vi "Save Report As PDF 2012 NIVerified.vi"(8 "error in (no error)":errorcluster, 10 "Data Set Name":string, 11 "Report file path":path=path "D:/Customer stuff/1944517 Tom Frei/test.xlsx") -> (0 "error out":errorcluster, 3 "Report Saved Path":path)   [LabVIEW 2020]
doc: "This VI demonstrates how to use ActiveX methods to save a Word or Excel report as a PDF."
uses:
  <vilib>/Utility/sysdir.llb/System Directory Type.ctl
  <vilib>/Utility/NIReport.llb/NI_report.lvclass
  <vilib>/Utility/NIReport.llb/Word/NI_Word.lvclass
  <vilib>/Utility/NIReport.llb/Excel/NI_Excel.lvclass
panel:
  # "Overview: Demonstrates how to use ActiveX methods to save a Word or Excel report as a PDF.  \nRequirements: LabVIEW 2012 (or compatible), Report Generation Toolkit\nInstructions: \n1. Browse for an existing Word or Excel document.\n2. Select the appropriate Report Type.\n3. Run the VI and it will save the document as a PDF as \"LabVIEW Save.pdf\" in the same folder as the original report."
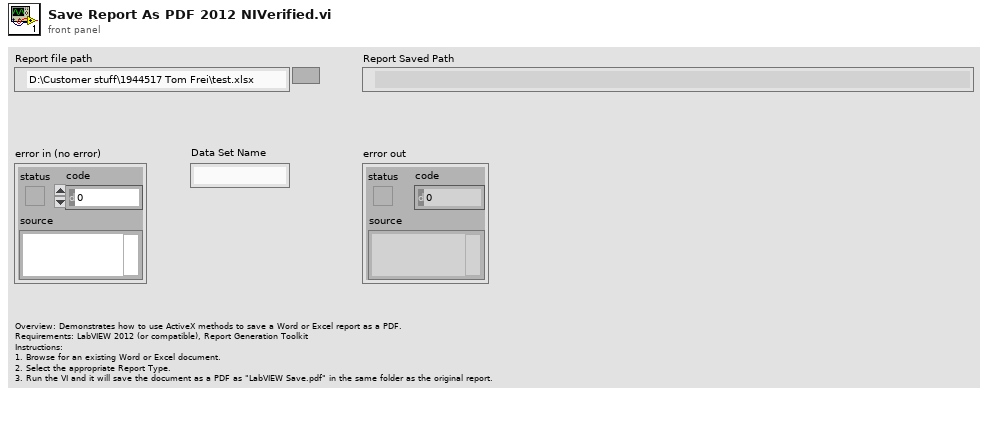
[diagram p1: front panel]
types:
  T1 = typedef "System Directory Type.ctl" = i32
  T2 = enum16{"Standard Report", "HTML", "Word", "Excel"}
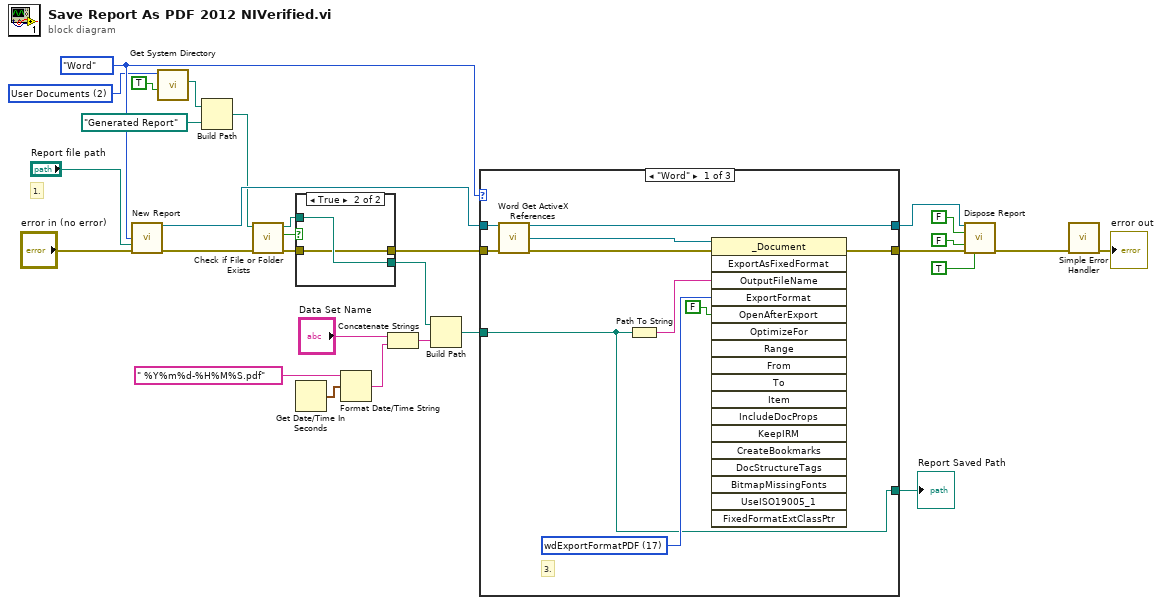
[diagram p0: block diagram]
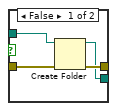
[diagram p2: hidden frame]
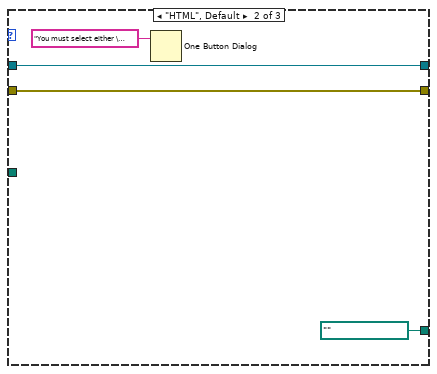
[diagram p3: hidden frame]
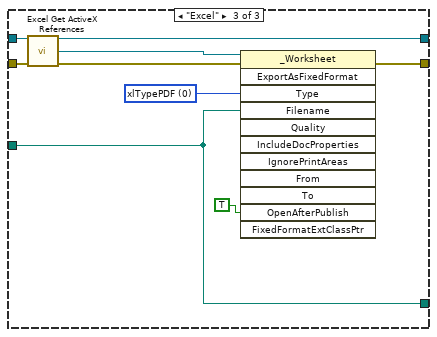
[diagram p4: hidden frame]
diagram:
  w21 = T1 2 items=["User Home"=0, "User Desktop"=1, "User Documents"=2, "User Application Data"=3, "User Preferences"=4, "User Temporary"=5, "Public Documents"=6, "Public Application Data"=7, "Public Preferences"=8, "Public Cache"=13, "System Core Libraries"=9, "System Installed Libraries"=10, "Application Files"=11, "Boot Volume Root"=12] ("system directory type")
  w27 = T2."Word" ("Report Type")
  # "1."
  n1 = call <vilib>:"New Report.vi"("report type"=w27, "template (empty)"="Report file path", "error in (no error)"="error in (no error)") -> ("report out"=w29:refnum<class "NI_report.lvclass">, "error out"=w7:errorcluster)  [unwired: 11 in]
  n2 = call <vilib>:"Get System Directory.vi"("create directory if not found? (F)"=TRUE, "system directory type"=w21) -> ("system directory"=w17:path)  [unwired: 9 in]
  n3 = Build Path(base path=w17, name or relative path=path "Generated Report") -> (appended path=w10:path)
  n4 = call <vilib>:"Check if File or Folder Exists.vi"("error in (no error)"=w7, "path"=w10) -> ("error out"=w6:errorcluster, "file or folder exists?"=w9:bool, "dup path"=w8:path)  [unwired: 7 in]
  n5 = case shown="True" w9 {
    tunnel: w8 -> [w33 w35]
    tunnel: w6 -> [w32 w34]
    tunnel: [w30 w35] -> w4
    tunnel: [w31 w34] -> w2
    frame False {
      n6 = Create Folder(path (use dialog)=w33, error in=w32) -> (created path=w30:path, error out=w31:errorcluster)  [unwired: 1 in, 1 out]
    }
    frame True {
    }
  }
  n7 = Get Date/Time In Seconds() -> (seconds since 1Jan1904=w19:timestamp)
  n8 = Format Date/Time String(time format string (%c)=" %Y%m%d-%H%M%S.pdf", seconds (now)=w19) -> (date/time string=w16:string)  [unwired: 1 in]
  n9 = Concatenate Strings("Data Set Name", w16) -> (w3:string)
  n10 = Build Path(base path=w4, name or relative path=w3) -> (appended path=w1:path)
  n11 = case shown="\"Word\"" w27 {
    tunnel: w29 -> [w45 w49 w57]
    tunnel: w1 -> [w36 _ w50]
    tunnel: [w44 w49 w55] -> w28
    tunnel: w2 -> [w40 w47 w54]
    tunnel: [w38 w47 w52] -> w26
    tunnel: [w36 path "" ("appended path") w50] -> w14
    frame "Word" {
      w41 = 17 items=["wdExportFormatPDF"=17, "wdExportFormatXPS"=18] ("ExportFormat")
      # "3."
      n12 = call <vilib>:"Word Get ActiveX References.vi"("report in"=w45, "error in (no error)"=w40) -> ("report out"=w44:refnum<class "NI_report.lvclass">, "Word._Document"=w43:refnum<k7>, "error out"=w39:errorcluster)  [unwired: 7 in, 4 out]
      n13 = Path To String(path=w36) -> (string=w42:string)
      n14 = invoke class="_Document" method="ExportAsFixedFormat"(reference=w43, error in=w39, "OutputFileName"=w42, "ExportFormat"=w41, "OpenAfterExport"=FALSE) -> (error out=w38:errorcluster)  [unwired: 13 in, 17 out]
    }
    frame "HTML", Default {
      n15 = One Button Dialog(message="You must select either \"Word\" or \"Excel\" as the Report Type.") -> ()  [unwired: 1 in, 1 out]
    }
    frame "Excel" {
      w51 = 0 items=["xlTypePDF", "xlTypeXPS"] ("Type")
      n16 = call <vilib>:"Excel Get ActiveX References.vi"("report in"=w57, "error in (no error)"=w54) -> ("report out"=w55:refnum<class "NI_report.lvclass">, "Excel._Worksheet"=w58:refnum<k7>, "error out"=w53:errorcluster)  [unwired: 7 in, 4 out]
      n17 = invoke class="_Worksheet" method="ExportAsFixedFormat"(reference=w58, error in=w53, "Type"=w51, "Filename"=w50, "OpenAfterPublish"=TRUE) -> (error out=w52:errorcluster)  [unwired: 7 in, 11 out]
    }
  }
  "Report Saved Path" <- w14
  n18 = call-dynamic "Dispose Report.vi"("report in"=w28, "wait until printing completed? (T)"=FALSE, "save changes? (F)"=FALSE, "error in (no error)"=w26, "close report? (T)"=TRUE) -> ("error out"=w25:errorcluster)  [unwired: 10 in]
  n19 = call <vilib>:"Simple Error Handler.vi"("error in (no error)"=w25) -> ("error out"=→"error out":errorcluster)  [unwired: 4 in, 4 out]
